vi "WSVCAP SHL Host TL I2C Write - Single Device.vi"(0 "Sub Address [U8]":u8=20 format="%.0x", 5 "Data Out [U8]":u8=20 format="%.0x", 11 "error in":errorcluster, 12 "DUT":T1, 13 "Device":T2, 14 "Log (T)":bool=TRUE) -> (15 "error out":errorcluster)   [LabVIEW 2012]
uses:
  Type Defs/WSVCAP SHL I2C Device Enum.ctl
  Type Defs/WSVCAP SHL DUT Number Enum.ctl
panel:
  out "C3 Data Out [U8]":u8[](array[numeric]) format="%.0x"
  out "Socket Mask [U32]":u32=1 format="%08x"
  out "C2 Data Out [U8]":u8[](array[numeric]) format="%.0x"
  out "C1 Data Out [U8]":u8[](array[numeric]) format="%.0x"
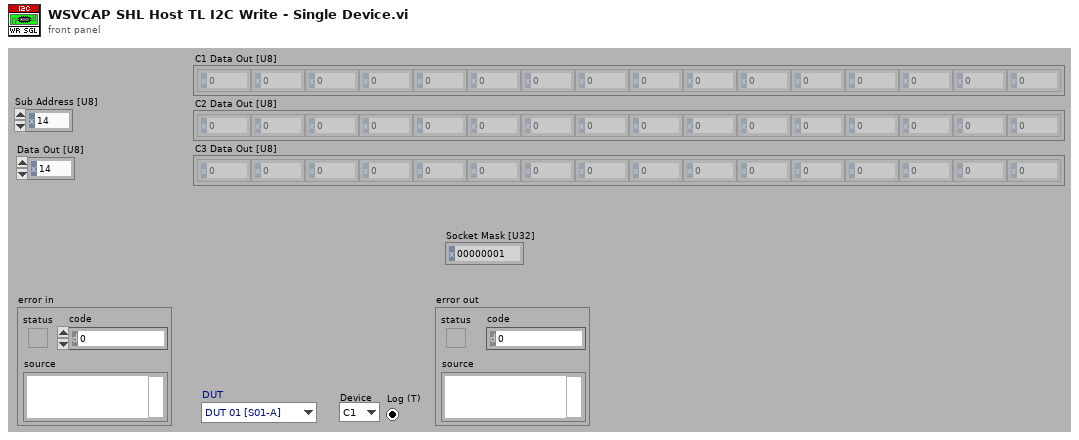
[diagram p1: front panel]
types:
  T1 = typedef "WSVCAP SHL DUT Number Enum.ctl" = enum16{"DUT 01 [S01-A]", "DUT 02 [S02-B]", "DUT 03 [S03-C]", "DUT 04 [S04-D]", "DUT 05 [S05-E]", "DUT 06 [S06-F]", "DUT 07 [S07-G]", "DUT 08 [S08-H]", "DUT 09 [S09-I]", "DUT 10 [S10-J]", "DUT 11 [S11-K]", "DUT 12 [S12-L]", "DUT 13 [S13-M]", "DUT 14 [S14-N]", "DUT 15 [S15-O]", "DUT 16 [S16-P]"}
  T2 = typedef "WSVCAP SHL I2C Device Enum.ctl" = enum16{"C1", "C2", "C3"}
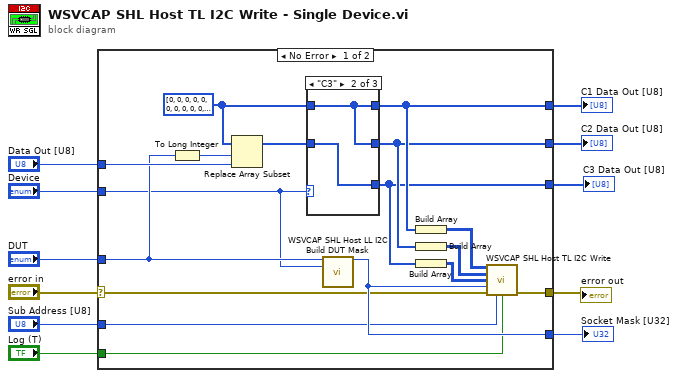
[diagram p0: block diagram]
diagram:
  n1 = case shown="No Error" "error in" {
    selector: "error in" -> [w17 w35]
    tunnel: [w28 w35] -> w11
    tunnel: "Sub Address [U8]" -> [w14 _]
    tunnel: "Data Out [U8]" -> [w27 _]
    tunnel: "Device" -> [w16 _]
    tunnel: [w21 _] -> w6
    tunnel: [w22 _] -> w5
    tunnel: "DUT" -> [w23 _]
    tunnel: [w18 _] -> w3
    tunnel: "Log (T)" -> [w15 _]
    tunnel: [w13 _] -> w1
    frame No Error {
      w25 = u8[] [0, 0, 0, 0, 0, 0, 0, 0, 0, 0, 0, 0, 0, 0, 0, 0] ("SPI Data Out")
      n2 = To Long Integer(number=w23) -> (32bit integer=w26:i32)
      n3 = Replace Array Subset(array=w25, new element=w27, index=w26) -> (w24:u8[])
      n4 = case shown="\"C3\"" w16 {
        tunnel: [w29 w31 w34] -> w22
        tunnel: w25 -> [w29 w31 w33]
        tunnel: [w30 w31 w33] -> w21
        tunnel: w24 -> [w30 w32 w34]
        tunnel: [w29 w32 w33] -> w13
        frame "C2" {
        }
        frame "C3" {
        }
        frame "C1" {
        }
      }
      n5 = call "WSVCAP SHL Host LL I2C Build DUT Mask.vi"("DUT"=w23, "Device"=w16) -> ("Socket Mask [U64]"=w18:u64)  [unwired: 11 in, 2 out]
      n6 = Build Array(w22) -> (w20:u8[][])
      n7 = Build Array(w21) -> (w19:u8[][])
      n8 = Build Array(w13) -> (w12:u8[][])
      n9 = call "WSVCAP SHL Host TL I2C Write.vi"("C1 Data Out"=w20, "C2 Data Out"=w19, "C3 Data Out"=w12, "Socket Mask [U64]"=w18, "error in"=w17, "Sub Address"=w14, "Log (T)"=w15) -> ("error out"=w28:errorcluster)  [unwired: 8 in]
    }
    frame Error {
    }
  }
  "error out" <- w11
  "C1 Data Out [U8]" <- w5
  "C2 Data Out [U8]" <- w6
  "Socket Mask [U32]" <- w3
  "C3 Data Out [U8]" <- w1
